vi "CPP-Inject_StackLoc.vi"() -> (5 "Plug in titles":string[](array[string]), 7 "Plug in values":string[](array[string]))   [LabVIEW 2015]
panel:
  # "Injects plugin values for stack location, either live, from ADAM server values, or in post, using raw data file metadata"
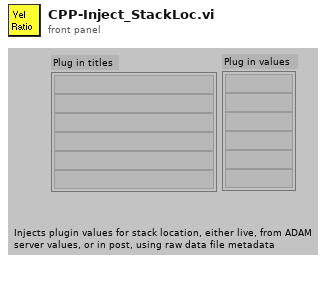
[diagram p1: front panel]
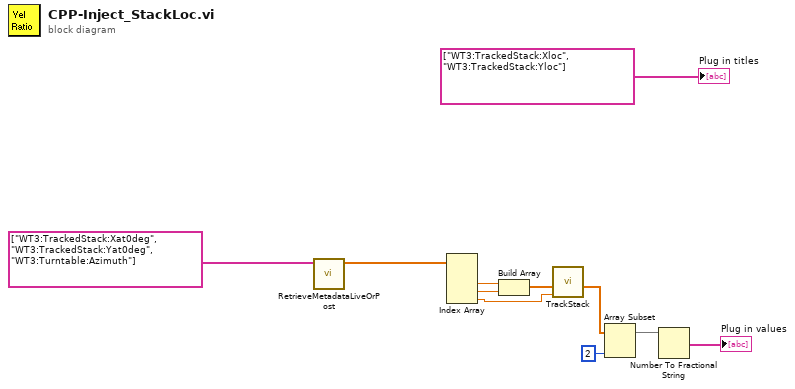
[diagram p0: block diagram]
diagram:
  n1 = call "RetrieveMetadataLiveOrPost.vi"("Array in"=string[] ["WT3:TrackedStack:Xat0deg", "WT3:TrackedStack:Yat0deg", "WT3:Turntable:Azimuth"]) -> ("Array out"=w1:dbl[])  [unwired: 10 in]
  n2 = Index Array(array=w1) -> (element #2=w4:dbl, element #3=w5:dbl, element #4=w2:dbl)  [unwired: 4 in, 1 out]
  n3 = Build Array(w4, w5) -> (w3:dbl[])
  n4 = call "TrackStack.vi"("WindDirection"=w2, "StackPosition (at 0deg)"=w3) -> ("CurrentStackPosition"=w7:sgl[])  [unwired: 8 in, 1 out]
  n5 = Array Subset(array=w7, length=2) -> (w8:sgl[])  [unwired: 1 in]
  n6 = Number To Fractional String(number=w8) -> (F-format string=→"Plug in values":string[])  [unwired: 3 in]
  "Plug in titles" <- string[] ["WT3:TrackedStack:Xloc", "WT3:TrackedStack:Yloc"]
